vi "UIStateExpr_Example2.vi"() -> ()   [LabVIEW 2017]
uses:
  RefManager/TagDB RefManager.lvlib
  <userlib>/_NEVSTOP/TagDB/TagDB.lvlib
  UIStateExpression/TagDB UIStateExpression.lvlib
panel:
  in  "aaa":string="aaaa"
  in  "toggle":bool
  in  "stop":bool
  in  "Boolean 0":bool
  in  "StateValue":i32
  in  "Boolean 5":bool
  in  "Boolean 4":bool
  in  "Boolean 3":bool
  in  "Boolean 2":bool
  in  "Boolean 1":bool
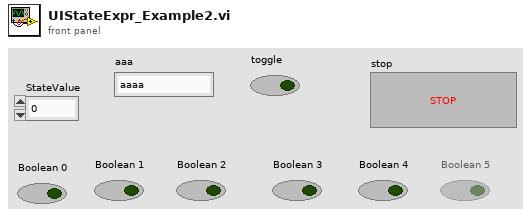
[diagram p1: front panel]
types:
  T1 = typedef "TagDB.lvlib/TagDB.ctl" = refnum<k1>
  T2 = typedef "TagDB RefManager.lvlib/RefMgr-Logic-State.ctl" = cluster{"StateName":string, "StateValue":i32, "Type":T3, "Calcs":cluster{"Tag":string, "Exp":string}[]}
  T3 = typedef "TagDB RefManager.lvlib/RefMgr-StateChangeType.ctl" = enum16{"0 - 进入", "1 - 等于", "2 - 退出"}
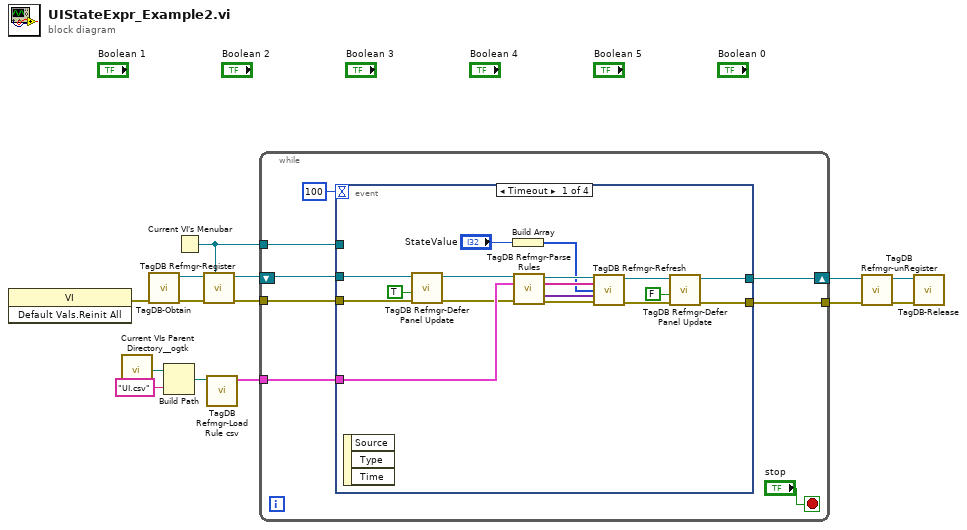
[diagram p0: block diagram]
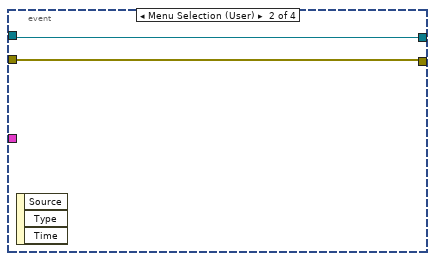
[diagram p2: hidden frame]
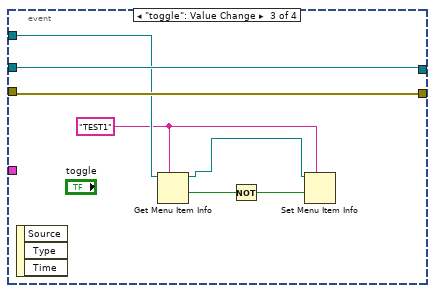
[diagram p3: hidden frame]
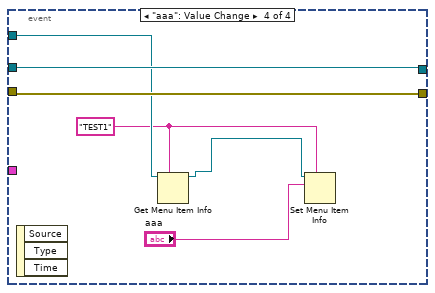
[diagram p4: hidden frame]
diagram:
  n1 = invoke class="VI" method="Default Vals.Reinit All"() -> (error out=w6:errorcluster)  [unwired: 3 in, 2 out]
  n2 = call <userlib>:"Current VIs Parent Directory__ogtk.vi"() -> ("Parent Directory (+ Relative)"=w3:path)  [unwired: 5 in]
  n3 = call <userlib>:"TagDB-Obtain.vi"("error in (no error)"=w6) -> ("error out"=w13:errorcluster, "TagDB"=w14:T1)  [unwired: 4 in, 1 out]
  n4 = Build Path(base path=w3, name or relative path="UI.csv") -> (appended path=w2:path)
  n5 = Current VI's Menubar() -> (w5:refnum<k9>)
  n6 = call "TagDB Refmgr-Register.vi"("menu reference"=w5, "error in (no error)"=w13, "TagDB in"=w14) -> ("error out"=w11:errorcluster, "TagDB out"=w12:T1)  [unwired: 6 in, 1 out]
  n7 = call "TagDB Refmgr-Load Rule csv.vi"("Path"=w2) -> ("Array 2"=w4:T2[])  [unwired: 9 in, 1 out]
  n8 = while {
    tunnel: w11 -> [w21]
    tunnel: w4 -> [w20]
    tunnel: [w17] -> w9
    shift-right: [w18] -> w10
    shift-left: w12 -> [w22]
    tunnel: w5 -> [w15]
    stop <- "stop" stop-if-true
    n9 = event shown="[0] Timeout" {
      selector: _ -> [_ _ _ _]
      dyn-events: _ -> [_ _ _ _]
      timeout: 100 -> [_ _ _ _]
      tunnel: w22 -> [w39 w41 w48 w54]
      tunnel: w21 -> [w28 w40 w47 w53]
      tunnel: w20 -> [w38 _ _ _]
      tunnel: [w29 w41 w48 w54] -> w18
      tunnel: [w25 w40 w47 w53] -> w17
      tunnel: w15 -> [_ _ w45 w51]
      event Timeout {
        n10 = event-data() -> ()  [unwired: 1 in, 3 out]
        n11 = call "TagDB Refmgr-Defer Panel Update.vi"("error in (no error)"=w28, "Defer Updates?"=TRUE, "TagDB in"=w39) -> ("error out"=w27:errorcluster, "TagDB out"=w30:T1)  [unwired: 7 in]
        n12 = Build Array("StateValue") -> (w32:i32[])
        n13 = call "TagDB Refmgr-Parse Rules.vi"("DB Ref"=w30, "Rules"=w38, "error in (no error)"=w27) -> ("DB Ref (dup)"=w37:T1, "StateNames"=w35:string[], "RulesMap"=w34:variant[], "error out"=w36:errorcluster)  [unwired: 9 in]
        n14 = call "TagDB Refmgr-Refresh.vi"("DB Ref"=w37, "StateName"=w35, "State"=w32, "RulesMap"=w34, "error in (no error)"=w36) -> ("DB Ref (dup)"=w31:T1, "error out"=w26:errorcluster)  [unwired: 9 in]
        n15 = call "TagDB Refmgr-Defer Panel Update.vi"("error in (no error)"=w26, "Defer Updates?"=FALSE, "TagDB in"=w31) -> ("error out"=w25:errorcluster, "TagDB out"=w29:T1)  [unwired: 7 in]
      }
      event Menu Selection (User) {
        n16 = event-data() -> ()  [unwired: 1 in, 3 out]
      }
      event "toggle": Value Change {
        w44 = "TEST1" ("item name")
        n17 = event-data() -> ()  [unwired: 1 in, 3 out]
        n18 = Get Menu Item Info(7:w44, 11:w45) -> (1:w43:bool, 3:w46:refnum<k9>)  [unwired: 1 in, 5 out]
        n19 = Not(x=w43) -> (.not. x?=w42:bool)
        n20 = Set Menu Item Info(7:w44, 9:w42, 11:w46) -> ()  [unwired: 4 in, 2 out]
      }
      event "aaa": Value Change {
        w50 = "TEST1" ("item name")
        n21 = event-data() -> ()  [unwired: 1 in, 3 out]
        n22 = Get Menu Item Info(7:w50, 11:w51) -> (3:w52:refnum<k9>)  [unwired: 1 in, 6 out]
        n23 = Set Menu Item Info(7:w50, 10:"aaa", 11:w52) -> ()  [unwired: 4 in, 2 out]
      }
    }
  }
  n24 = call "TagDB Refmgr-unRegister.vi"("error in (no error)"=w9, "TagDB in"=w10) -> ("error out"=w8:errorcluster, "TagDB out"=w7:T1)  [unwired: 8 in]
  n25 = call <userlib>:"TagDB-Release.vi"("error in (no error)"=w8, "TagDB"=w7) -> ()  [unwired: 9 in, 1 out]
